vi "Open API Reference.vi"(8 "error in (no error)":errorcluster) -> (0 "error out":errorcluster, 3 "Execution API Out":refnum<class "Execution API.lvclass">)   [LabVIEW 2020, in "Execution API.lvclass"]
doc: "Initializes the API and obtains a reference. The reference should be closed using the Close API Reference.vi when it is no longer needed."
uses:
  Execution API.lvclass
  Core/Result/Result.ctl
  Core/Result/Status.ctl
  Core/Result/Type.ctl
  Execution API.lvclass/Execution API.ctl
  Framework/Single Thread Test Runner/Single Thread Test Runner.lvclass
  C:/git/astemes-lunit/source/Framework/Test Runner/Test Runner.lvclass
  Core/Result/Result.lvlib
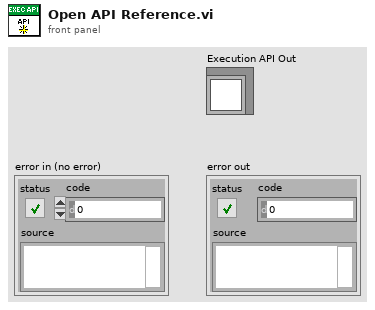
[diagram p1: front panel]
types:
  T1 = typedef "Result.lvlib/Result.ctl" = cluster{"Name":string, "Message":string, "Description":string, "Status":T2, "Result Type":T3, "Execution Time":dbl}
  T2 = typedef "Result.lvlib/Status.ctl" = enum16{"", "Passed", "Failed", "Error", "Skipped", "Setup Error", "Broken", "Teardown Error"}
  T3 = typedef "Result.lvlib/Type.ctl" = enum16{"Test Case", "Test Suite", "Test Run", "Pass", "Fail", "Skip", "Pass if", "Fail if", "Pass if Error", "Fail if Error", "Pass if Equal", "Fail if Equal"}
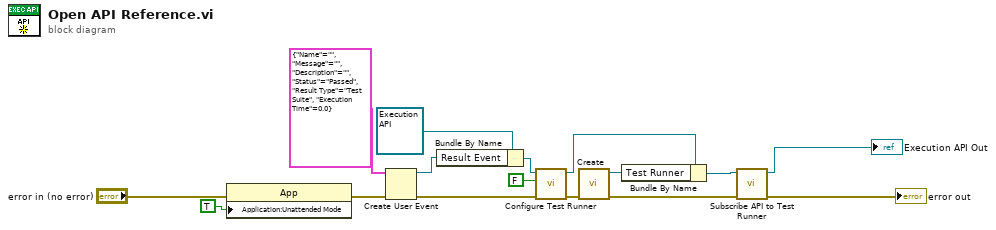
[diagram p0: block diagram]
diagram:
  n1 = property class="App"(error in="error in (no error)", "Application:Unattended Mode"=TRUE) -> (error out=w5:errorcluster)  [unwired: 1 in, 1 out]
  n2 = Create User Event(user event datatype=T1 {"Name"="", "Message"="", "Description"="", "Status"=enum."Passed", "Result Type"=enum."Test Suite", "Execution Time"=0.0} ("Result"), error in=w5) -> (user event=w8:refnum<user-event>, error out=w7:errorcluster)
  n3 = Bundle By Name(cluster=refnum<class "Execution API.lvclass"> refnum ("LUnit API.lvclass"), "Result Event"=w8) -> (w9:refnum<class "Execution API.lvclass">)
  n4 = call "Configure Test Runner.vi"("error in (no error)"=w7, "Run Tests In Parallel?"=FALSE, "Execution API In"=w9) -> ("error out"=w11:errorcluster, "Execution API Out"=w15:refnum<class "Execution API.lvclass">)  [unwired: 7 in]
  n5 = call "Create.vi"("error in (no error)"=w11) -> ("error out"=w12:errorcluster, "Single Thread Test Runner out"=w13:refnum<class "Single Thread Test Runner.lvclass">)  [unwired: 9 in]
  n6 = Bundle By Name(cluster=w15, "Test Runner"=w13) -> (w2:refnum<class "Execution API.lvclass">)
  n7 = call "Subscribe API to Test Runner.vi"("error in (no error)"=w12, "Execution API In"=w2) -> ("error out"=→"error out":errorcluster, "Execution API Out"=→"Execution API Out":refnum<class "Execution API.lvclass">)  [unwired: 8 in]
